vi "FuncImg-Initialise Controls.vi"   [LabVIEW 2013]
uses:
  Global variables/gl_Functional Imaging-Global variables.vi
types:
  T1 = typedef "Functional Imging UI Refs.ctl" = cluster{"Menu ref":refnum<k9>, "Image control":refnum<vi>, "VI ref":refnum<vi>, "XGrapher":refnum<vi>, "Smoothing":refnum<vi>, "POI Averaging":refnum<vi>, "Normalize":refnum<vi>, "POI data points in each trial":refnum<vi>, "Channel":refnum<vi>, "Experiment data folder path":refnum<vi>, "[ROI vis]":refnum<vi>, "[Groups] visbl":T2, "Group Name":refnum<vi>, "POI index":refnum<vi>, "Trial No.":refnum<vi>, "Intensity Zoom":refnum<vi>, "Trial Cursor Enabled":refnum<vi>, "Number of Trials (ind 1)":refnum<vi>, "Number of Trials (ind 2)":refnum<vi>, "MiniScans Available":refnum<vi>, "POI Available":refnum<vi>, "Defer graph updates":refnum<vi>, "Waveform selector":refnum<vi>, "#of selected POI":refnum<vi>, "#of selected MiniScans":refnum<vi>, "#of selected groups":refnum<vi>, "Max Z-Projection":refnum<vi>, "Z-Plane Selector":refnum<vi>, "Index of miniscan point to visualise":refnum<vi>, "ROI vis. mode":refnum<vi>, "Total # of points":refnum<vi>, "Index of group clicked on":refnum<vi>, "Pane 1":refnum<vi>, "Pane 2":refnum<vi>, "Pane 3":refnum<vi>, "Pane 4":refnum<vi>, "Pane 5":refnum<vi>, "Pane 6":refnum<vi>, "Deselect all ROI":refnum<vi>, "Deselect all groups":refnum<vi>}
  T2 = typedef "Groups array referecne.ctl" = refnum<vi>
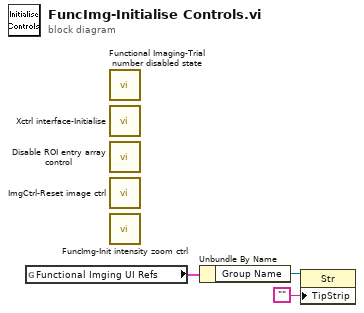
[diagram p0: block diagram]
diagram:
  n1 = global read "gl_Functional Imaging-Global variables.vi" "Functional Imging UI Refs"() -> (w3:T1)
  n2 = call "Functional Imaging-Trial number disabled state.vi"() -> ()  [unwired: 12 in]
  n3 = call "Xctrl interface-Initialise.vi"() -> ()  [unwired: 11 in, 1 out]
  n4 = call "Disable ROI entry array control.vi"() -> ()  [unwired: 12 in]
  n5 = call "ImgCtrl-Reset image ctrl.vi"() -> ()  [unwired: 11 in, 1 out]
  n6 = call "FuncImg-Init intensity zoom ctrl.vi"() -> ()  [unwired: 12 in]
  n7 = Unbundle By Name(w3) -> ("Group Name"=w2:refnum<vi>)
  n8 = property class="Str"(reference=w2, "TipStrip"="" ("Tip Strip")) -> ()  [unwired: 1 in, 2 out]
